vi "Get ID.vi"(8 "error in (no error)":errorcluster, 11 "Execution in":refnum<class "Execution.lvclass">) -> (0 "error out":errorcluster, 2 "Id":i32, 3 "Execution out":refnum<class "Execution.lvclass">)   [LabVIEW 2020, in "TSnax.lvlib" / "Execution.lvclass"]
uses:
  Execution.lvclass
  Execution.lvclass/Execution.ctl
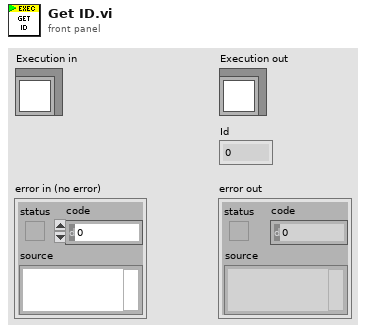
[diagram p1: front panel]
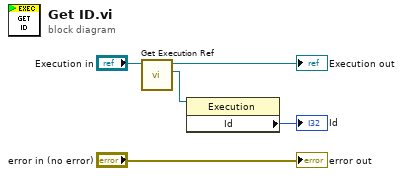
[diagram p0: block diagram]
diagram:
  n1 = call "Get Execution Ref.vi"("Execution in"="Execution in") -> ("Execution Ref"=w3:refnum<k7>, "Execution out"=→"Execution out":refnum<class "Execution.lvclass">)  [unwired: 8 in, 1 out]
  n2 = property class="Execution"(reference=w3) -> ("Id"=→"Id":i32)  [unwired: 1 in, 2 out]
  "error out" <- "error in (no error)"
